vi "Frequency Weighting for Power.vi"(0 "power spectrum [EUrms^2]":dbl[](array[numeric]) format="%.2f", 1 "df [Hz]":dbl format="%.2f", 2 "frequency weighting":T4(ring), 3 "channel info":T1={"sensor sensitivity [mV/EU]"=1000.0, "engineering units"=1, "dB reference [EU]"=1.0, "custom label"="EU", "weighting filter"=0, "pregain [dB]"=0.0} {"pregain [dB]" format="%.2f"; "weighting filter" items=["Linear", "A-weighting", "B-weighting", "C-weighting", "ITU-R 468-4", "Dolby", "CCITT", "C-message"]; "dB reference [EU]" format="%^.1e"; "engineering units" items=["custom..."=0, "V"=1, "A"=21, "Pa"=2, "N"=20, "g"=3, "m/s^2"=4, "m/s"=5, "m"=6, "mm/s"=12, "mm"=13, "microns/s"=14, "microns"=15, "in/s^2"=7, "in/s"=8, "in"=9, "mils/s"=10, "mils"=11, "rad/s^2"=16, "rad/s"=17, "rad"=18, "strain"=19]; "sensor sensitivity [mV/EU]" format="%.2f"}, 4 "dB On (F)":bool) -> (5 "frequency weighted power [EUrms^2]":dbl[](array[numeric]) format="%.2f", 6 "unit label":string, 7 "weighting conflict":bool)   [LabVIEW 2017]
uses:
  <vilib>/addons/Sound and Vibration/compatibility/Controls/svl_Channel Info.ctl
  <vilib>/addons/Sound and Vibration/compatibility/Controls/svl_Engineering Units Text Ring.ctl
  <vilib>/addons/Sound and Vibration/compatibility/Controls/svl_Weighting Filter Text Ring.ctl
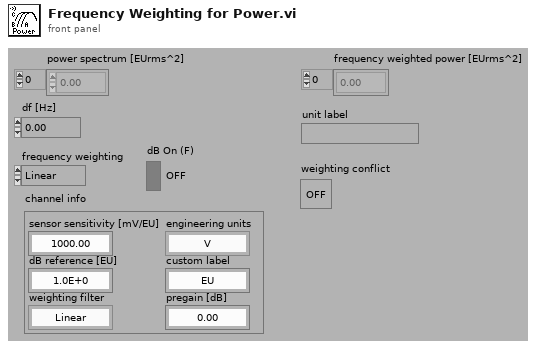
[diagram p1: front panel]
types:
  T1 = typedef "svl_Channel Info.ctl" = cluster{"sensor sensitivity [mV/EU]":dbl, "engineering units":T2, "dB reference [EU]":dbl, "custom label":string, "weighting filter":T3, "pregain [dB]":dbl}
  T2 = typedef "svl_Engineering Units Text Ring.ctl" = u16
  T3 = typedef "svl_Weighting Filter Text Ring.ctl" = u16
  T4 = enum16{"Linear", "A-weighting", "B-weighting", "C-weighting"}
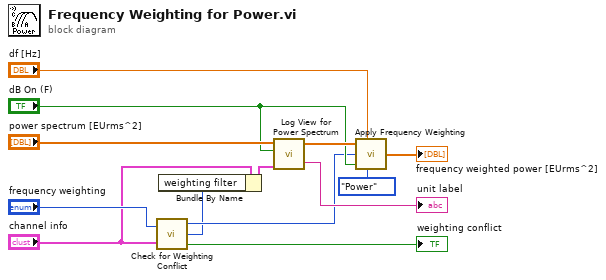
[diagram p0: block diagram]
diagram:
  n1 = call <vilib>:"Check for Weighting Conflict.vi"("weighting filter"="frequency weighting", "channel info"="channel info") -> ("weighting to apply"=w4:T4, "weighting units"=w1:T4, "weighting conflict"=→"weighting conflict":bool)
  n2 = Bundle By Name(cluster="channel info", "weighting filter"=w1) -> (w2:T1)
  n3 = call <vilib>:"Log View for Power Spectrum.vi"("channel info"=w2, "dB On (T)"="dB On (F)", "power spectrum [EU^2 rms]"="power spectrum [EUrms^2]") -> ("unit label"=→"unit label":string, "log view power spectrum [dB EU]"=w8:dbl[])  [unwired: 1 in]
  n4 = call <vilib>:"Apply Frequency Weighting.vi"("spectrum"=w8, "df [Hz]"="df [Hz]", "weighting filter"=w4, "dB On (T)"="dB On (F)", "spectrum type"=enum16{"Power", "Amplitude"}."Power") -> ("frequency weighted spectrum"=→"frequency weighted power [EUrms^2]":dbl[])
